vi "Task04.vi"() -> ()   [LabVIEW 2017]
panel:
  out "Slide":u8(slide) scale=0.0..255.0
  out "Meter":dbl(knob) scale=0.0..255.0
  out "Thermometer":dbl(slide) scale=0.0..255.0
  out "Numeric":dbl
  in  "stop":bool
  in  "Switch Array":bool[](array[boolean])
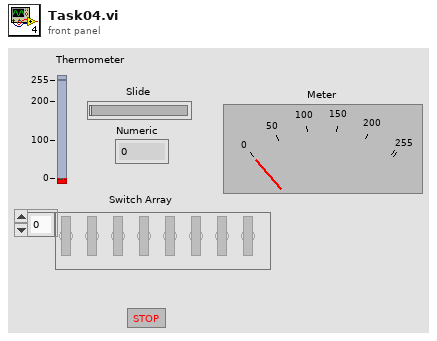
[diagram p1: front panel]
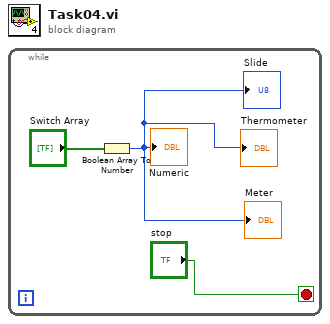
[diagram p0: block diagram]
diagram:
  n1 = while {
    stop <- "stop" stop-if-true
    n2 = Boolean Array To Number(Boolean array="Switch Array") -> (number=→"Numeric" →"Thermometer" →"Meter" →"Slide":u32)
  }
